vi "Generator_c.vi"(0 "Stop":bool caption="Start/Stop") -> (4 "Generated_Data":dbl caption="Generated Data")   [LabVIEW 2023]
doc: "This VI continuously generate Data and push it to the Acquisition VI.\nTransfer of thet data happens under Queue LV2."
uses:
  Type_Def/Operation_Queue.ctl
  <vilib>/numeric/Random Number (Range) DBL.vi
panel:
  out "Error_Out":errorcluster
  in  "Error_In":errorcluster
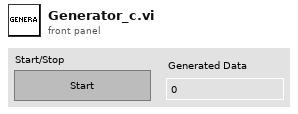
[diagram p1: front panel]
types:
  T1 = typedef "Operation_Queue.ctl" = enum16{"Initialize", "Enqueue", "Dequeue", "Sum"}
  T2 = enum16{"Left Button", "Center Button", "Right Button", "Window Close"}
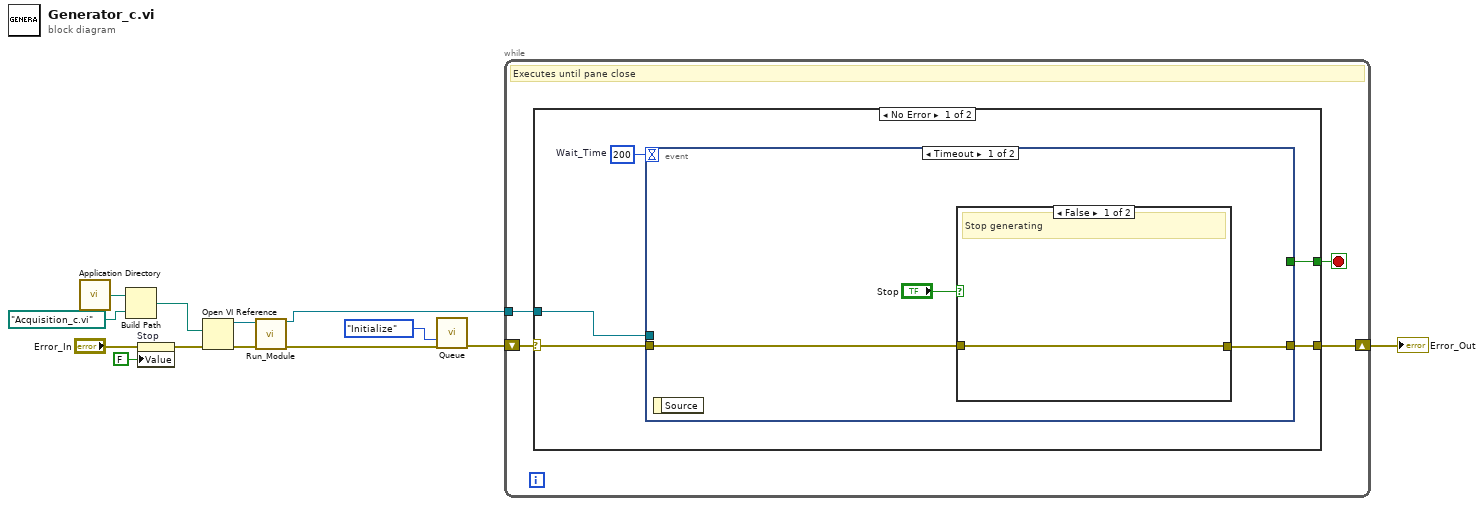
[diagram p0: block diagram]
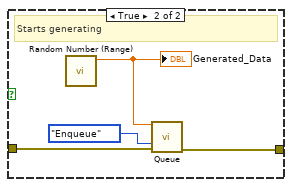
[diagram p2: hidden frame]
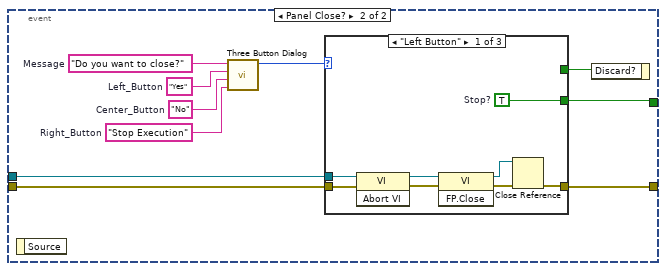
[diagram p3: hidden frame]
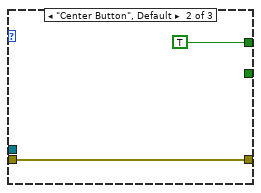
[diagram p4: hidden frame]
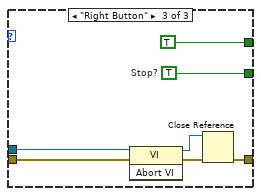
[diagram p5: hidden frame]
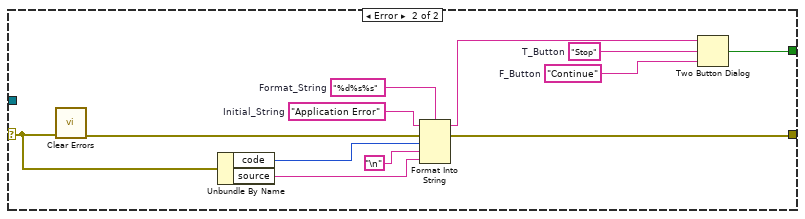
[diagram p6: hidden frame]
diagram:
  n1 = call <vilib>:"Application Directory.vi"() -> ("Application Directory"=w12:path)
  n2 = Build Path(base path=w12, name or relative path=path "Acquisition_c.vi") -> (appended path=w11:path)
  n3 = property on="Stop" class="Bool (strict)"(error in="Error_In", "Value"=FALSE ("Stop")) -> (error out=w4:errorcluster)  [unwired: 1 in, 1 out]
  n4 = Open VI Reference(vi path=w11, error in (no error)=w4) -> (vi reference=w5:refnum<vi>, error out=w6:errorcluster)  [unwired: 4 in]
  n5 = call "Run_Module.vi"("VI_In"=w5, "Error_In"=w6) -> ("VI_Out"=w7:refnum<vi>, "Error_Out"=w1:errorcluster)  [unwired: 12 in]
  n6 = call "Queue.vi"("Operation"=Operation_Queue."Initialize" ("Operation_Queue"), "Error_In"=w1) -> ("Error_Out"=w9:errorcluster)  [unwired: 9 in, 4 out]
  n7 = while {
    shift-right: [w15] -> w8
    shift-left: w9 -> [w16]
    tunnel: w7 -> [w14]
    stop <- w17 stop-if-true
    # "Executes until pane close"
    n8 = case shown="No Error" w16 {
      selector: w16 -> [w20 w60]
      tunnel: [w21 w58] -> w17
      tunnel: [w19 w59] -> w15
      tunnel: w14 -> [w18 _]
      frame No Error {
        w22 = 200  # Wait_Time
        n9 = event shown="[0] Timeout" {
          selector: _ -> [_ _]
          dyn-events: _ -> [_ _]
          timeout: w22 -> [_ _]
          tunnel: [_ w35] -> w21
          tunnel: w20 -> [w23 w34]
          tunnel: [w24 w32] -> w19
          tunnel: w18 -> [_ w33]
          event Timeout {
            n10 = event-data() -> ()  [unwired: 1 in, 1 out]
            n11 = case shown="False" "Stop" {
              tunnel: w23 -> [w26 w27]
              tunnel: [w26 w30] -> w24
              frame False {
                # "Stop generating"
              }
              frame True {
                # "Starts generating"
                n12 = call-poly <vilib>:"Random Number (Range).vi"() -> ("number"=w29:dbl)  [unwired: 11 in]
                "Generated_Data" <- w29
                n13 = call "Queue.vi"("Element_In"=w29, "Operation"=Operation_Queue."Enqueue" ("Operation_Queue"), "Error_In"=w27) -> ("Error_Out"=w30:errorcluster)  [unwired: 8 in, 4 out]
              }
            }
          }
          event Panel Close? {
            w37 = "Stop Execution"  # Right_Button
            w38 = "No"  # Center_Button
            w39 = "Yes"  # Left_Button
            w40 = "Do you want to close?"  # Message
            n14 = event-data() -> ()  [unwired: 1 in, 1 out]
            n15 = call <vilib>:"Three Button Dialog.vi"("Right Button Text (\"Cancel\")"=w37, "Center Button Text (\"No\")"=w38, "Left Button Text (\"Yes\")"=w39, "message"=w40) -> ("Which Button?"=w31:T2)  [unwired: 7 in]
            n16 = case shown="\"Left Button\"" w31 {
              tunnel: [_ TRUE ("Discard?") TRUE ("Discard?")] -> w36
              tunnel: [w48 _ w57] -> w35
              tunnel: w34 -> [w43 w49 w53]
              tunnel: w33 -> [w44 _ w52]
              tunnel: [w41 w49 w51] -> w32
              frame "Left Button" {
                w48 = TRUE  # Stop?
                n17 = invoke class="VI" method="Abort VI"(reference=w44, error in=w43) -> (reference out=w45:refnum<vi>, error out=w42:errorcluster)  [unwired: 1 in, 1 out]
                n18 = invoke class="VI" method="FP.Close"(reference=w45, error in=w42) -> (reference out=w47:refnum<vi>, error out=w46:errorcluster)  [unwired: 1 in, 1 out]
                n19 = Close Reference(reference=w47, error in (no error)=w46) -> (error out=w41:errorcluster)
              }
              frame "Center Button", Default {
              }
              frame "Right Button" {
                w57 = TRUE  # Stop?
                n20 = invoke class="VI" method="Abort VI"(reference=w52, error in=w53) -> (reference out=w55:refnum<vi>, error out=w54:errorcluster)  [unwired: 1 in, 1 out]
                n21 = Close Reference(reference=w55, error in (no error)=w54) -> (error out=w51:errorcluster)
              }
            }
            n22 = event-data ("Event Filter Node")("Discard?"=w36) -> ()  [unwired: 1 in, 1 out]
          }
        }
      }
      frame Error {
        w65 = "%d%s%s"  # Format_String
        w66 = "Application Error"  # Initial_String
        w67 = "Stop"  # T_Button
        w68 = "Continue"  # F_Button
        n23 = call <vilib>:"Clear Errors.vi"("error in (no error)"=w60) -> ("error out"=w63:errorcluster)  [unwired: 5 in, 1 out]
        n24 = Unbundle By Name(w60) -> ("code"=w62:i32, "source"=w61:string)
        n25 = Format Into String(format string=w65, initial string=w66, error in=w63, w62, "\n", w61) -> (resulting string=w69:string, error out=w59:errorcluster)
        n26 = Two Button Dialog(message=w69, 1:w68, 2:w67) -> (T button?=w58:bool)
      }
    }
  }
  "Error_Out" <- w8
